vi "loadDataNodeBegin.vi"(8 "error in (no error)":errorcluster, 10 "XML Refnum in":refnum<file>, 11 "FPGADMAChannelData in":refnum<class "FPGADMAChannelData.lvclass">) -> (0 "error out":errorcluster, 2 "XML Refnum out":refnum<file>, 3 "FPGADMAChannelData out":refnum<class "FPGADMAChannelData.lvclass">)   [LabVIEW 2013, in "FPGADMAChannelData.lvclass"]
doc: "Part of the file loading process. Occurs at the beginning of a node being loaded. Loads the common xceDataNode data name and description."
uses:
  FPGADMAChannelData.lvclass
  FPGADMAChannelData.lvclass/FPGADMAChannelData.ctl
  xCE/xceNode/xceNode.lvclass
  XML Parser/XML Parser.lvclass
panel:
  out "text":string[](array[string])
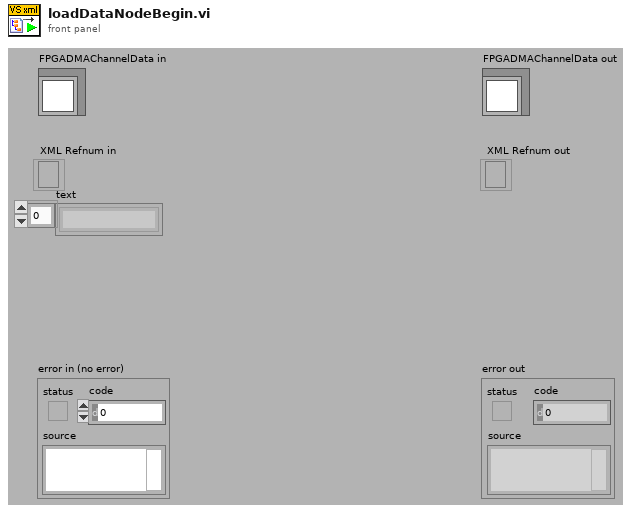
[diagram p1: front panel]
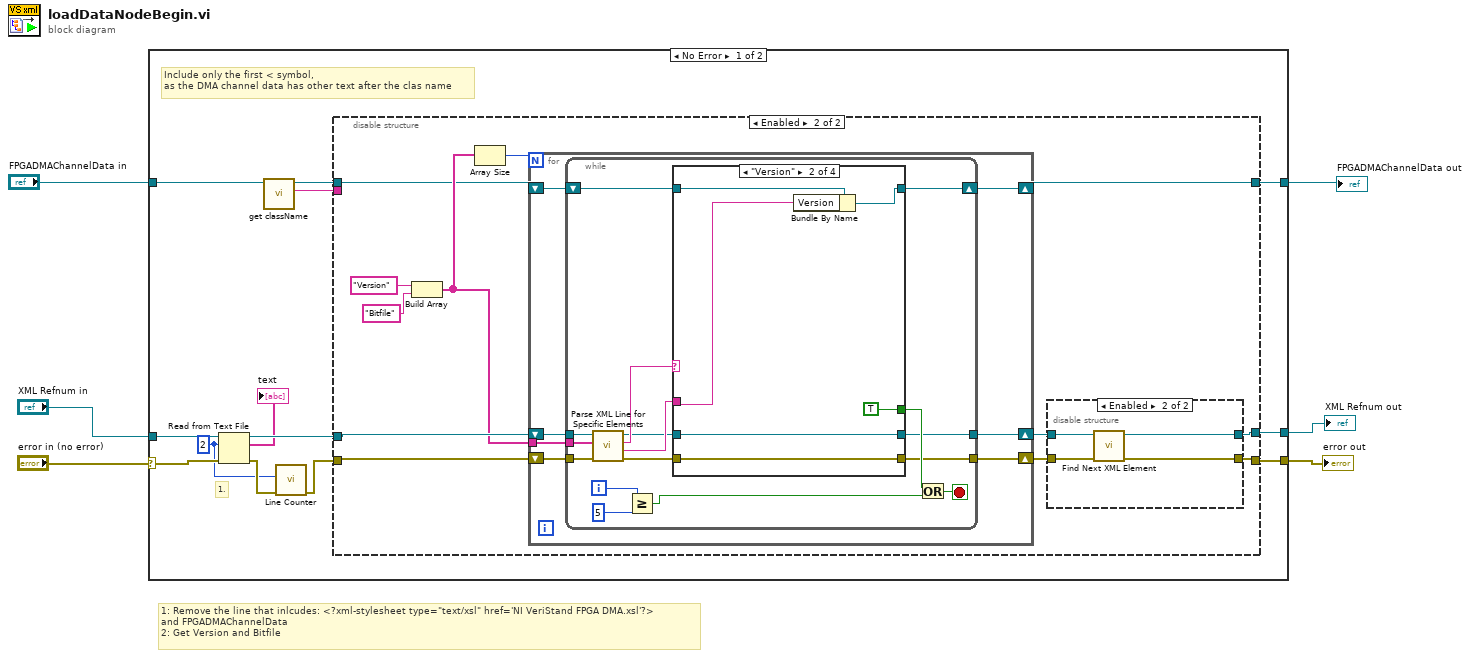
[diagram p0: block diagram]
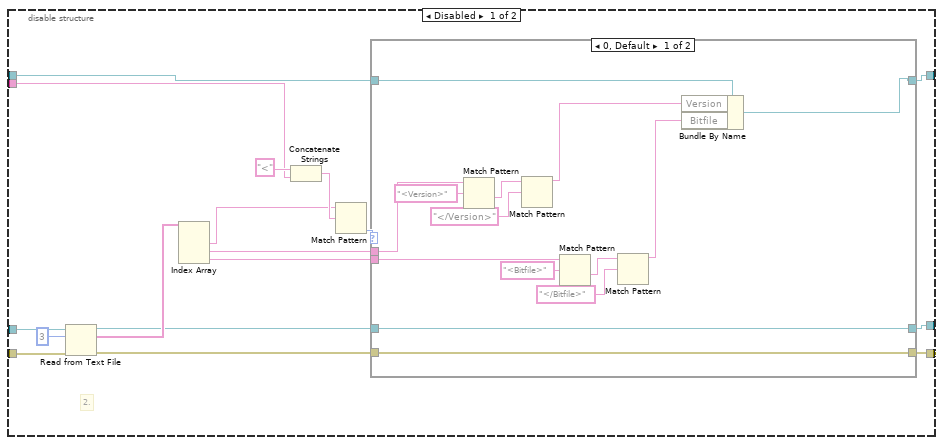
[diagram p2: hidden frame]
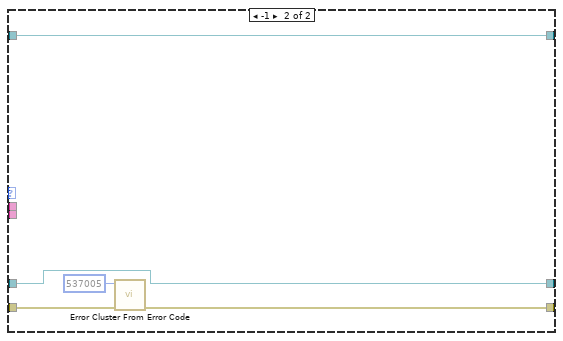
[diagram p3: hidden frame]
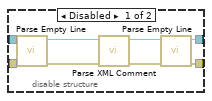
[diagram p4: hidden frame]
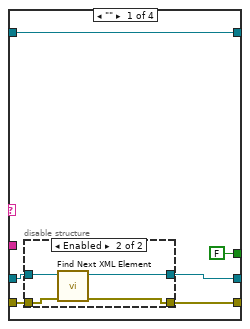
[diagram p5: hidden frame]
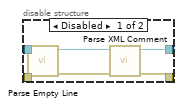
[diagram p6: hidden frame]
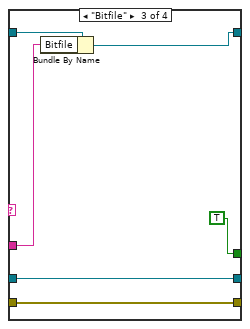
[diagram p7: hidden frame]
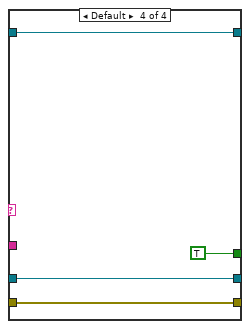
[diagram p8: hidden frame]
diagram:
  # "1: Remove the line that inlcudes: <?xml-stylesheet type=\"text/xsl\" href='NI VeriStand FPGA DMA.xsl'?>\nand FPGADMAChannelData \n2: Get Version and Bitfile"
  n1 = case shown="No Error" "error in (no error)" {
    selector: "error in (no error)" -> [w13 w137]
    tunnel: [w18 w137] -> w3
    tunnel: [w15 w136] -> w2
    tunnel: [w16 w135] -> w1
    tunnel: "FPGADMAChannelData in" -> [w14 w136]
    tunnel: "XML Refnum in" -> [w12 w135]
    frame No Error {
      w7 = 2 ("count")
      # "Include only the first < symbol,\nas the DMA channel data has other text after the clas name"
      # "1."
      n2 = Read from Text File(file (use dialog)=w12, count=w7, error in=w13) -> (refnum out=w11:refnum<file>, text=→"text":string[], error out=w9:errorcluster)  [unwired: 1 in, 1 out]
      n3 = call "get className.vi"("xceNode in"=w14) -> ("Class name"=w19:string, "xceNode out"=w17:refnum<class "FPGADMAChannelData.lvclass">)  [unwired: 8 in, 1 out]
      n4 = call "Line Counter.vi"("error in (no error)"=w9, "# of lines to increment (1)"=w7) -> ("error out"=w8:errorcluster)  [unwired: 8 in, 1 out]
      n5 = disable-structure shown="Enabled" {
        disable-tunnel: w19 -> [w33 _]
        disable-tunnel: [w28 w56] -> w18
        disable-tunnel: w17 -> [w27 w61]
        disable-tunnel: [w23 w57] -> w16
        disable-tunnel: [w22 w60] -> w15
        disable-tunnel: w11 -> [w21 w65]
        disable-tunnel: w8 -> [w20 w64]
        frame Disabled {
          # "2."
          n6 = Read from Text File(file (use dialog)=w21, count=3, error in=w20) -> (refnum out=w24:refnum<file>, text=w35:string[], error out=w30:errorcluster)  [unwired: 1 in, 1 out]
          n7 = Index Array(array=w35) -> (element #1=w31:string, element #2=w26:string, element #3=w25:string)  [unwired: 3 in]
          n8 = Concatenate Strings("<", w33) -> (w32:string)
          n9 = Match Pattern(string=w31, regular expression=w32) -> (offset past match=w29:i32)  [unwired: 1 in, 3 out]
          n10 = case shown="0, Default" w29 {
            tunnel: w30 -> [w50 w55]
            tunnel: [w50 w54] -> w28
            tunnel: w27 -> [w38 w51]
            tunnel: w26 -> [w48 _]
            tunnel: w25 -> [w40 _]
            tunnel: w24 -> [w49 w52]
            tunnel: [w49 w52] -> w23
            tunnel: [w37 w51] -> w22
            frame 0, Default {
              n11 = Match Pattern(string=w48, regular expression="<Version>") -> (after substring=w46:string)  [unwired: 1 in, 3 out]
              n12 = Match Pattern(string=w46, regular expression="</Version>") -> (before substring=w44:string)  [unwired: 1 in, 3 out]
              n13 = Match Pattern(string=w40, regular expression="<Bitfile>") -> (after substring=w42:string)  [unwired: 1 in, 3 out]
              n14 = Match Pattern(string=w42, regular expression="</Bitfile>") -> (before substring=w39:string)  [unwired: 1 in, 3 out]
              n15 = Bundle By Name(cluster=w38, "Version"=w44, "Bitfile"=w39) -> (w37:refnum<class "FPGADMAChannelData.lvclass">)
            }
            frame -1 {
              n16 = call <vilib>:"Error Cluster From Error Code.vi"("error in (no error)"=w55, "error code (0)"=537005) -> ("error out"=w54:errorcluster)  [unwired: 7 in]
            }
          }
        }
        frame Enabled {
          n17 = Build Array("Version" ("regular expression"), "Bitfile" ("regular expression")) -> (w63:string[])
          n18 = Array Size(array=w63) -> (size(s)=w62:i32)
          n19 = for {
            N: w62 -> [_]
            tunnel: w63 -> [w86]
            shift-right: [w81] -> w60
            shift-left: w61 -> [w83]
            shift-right: [w82] -> w59
            shift-left: w65 -> [w85]
            shift-right: [w80] -> w58
            shift-left: w64 -> [w84]
            n20 = while {
              tunnel: w86 -> [w102]
              tunnel: w85 -> [w101]
              tunnel: w84 -> [w100]
              shift-right: [w95] -> w81
              shift-left: w83 -> [w97]
              tunnel: [w87] -> w82
              tunnel: [w88] -> w80
              i -> [w99]
              stop <- w92 stop-if-true
              n21 = call "Parse XML Line for Specific Elements.vi"("error in (no error)"=w100, "Elements"=w102, "XML Refnum in"=w101) -> ("error out"=w89:errorcluster, "Value"=w91:string, "Element Name"=w96:string, "XML Refnum out"=w90:refnum<file>)  [unwired: 4 in, 1 out]
              n22 = Greater Or Equal?(x=w99, y=5) -> (x >= y?=w93:bool)
              n23 = case shown="\"Version\"" w96 {
                tunnel: w97 -> [w108 w124 w130 w134]
                tunnel: [w108 w123 w129 w134] -> w95
                tunnel: [FALSE TRUE TRUE TRUE] -> w94
                tunnel: w91 -> [_ w122 w128 _]
                tunnel: w90 -> [w107 w120 w126 w132]
                tunnel: w89 -> [w106 w119 w125 w131]
                tunnel: [w105 w119 w125 w131] -> w88
                tunnel: [w104 w120 w126 w132] -> w87
                frame "" {
                  n24 = disable-structure shown="Enabled" {
                    disable-tunnel: w107 -> [w114 w118]
                    disable-tunnel: w106 -> [w113 w117]
                    disable-tunnel: [w110 w116] -> w105
                    disable-tunnel: [w109 w115] -> w104
                    frame Disabled {
                      n25 = call "Parse Empty Line.vi"("error in (no error)"=w113, "XML Refnum in"=w114) -> ("error out"=w111:errorcluster, "XML Refnum out"=w112:refnum<file>)  [unwired: 7 in, 1 out]
                      n26 = call "Parse XML Comment.vi"("error in (no error)"=w111, "XML Refnum in"=w112) -> ("error out"=w110:errorcluster, "XML Refnum out"=w109:refnum<file>)  [unwired: 6 in, 2 out]
                    }
                    frame Enabled {
                      n27 = call "Find Next XML Element.vi"("error in (no error)"=w117, "XML Fine In"=w118) -> ("error out"=w116:errorcluster, "XML Fine Out"=w115:refnum<file>)  [unwired: 7 in, 1 out]
                    }
                  }
                }
                frame "Version" {
                  n28 = Bundle By Name(cluster=w124, "Version"=w122) -> (w123:refnum<class "FPGADMAChannelData.lvclass">)
                }
                frame "Bitfile" {
                  n29 = Bundle By Name(cluster=w130, "Bitfile"=w128) -> (w129:refnum<class "FPGADMAChannelData.lvclass">)
                }
                frame Default {
                }
              }
              n30 = Or(x=w94, y=w93) -> (x .or. y?=w92:bool)
            }
          }
          n31 = disable-structure shown="Enabled" {
            disable-tunnel: w59 -> [w71 w79]
            disable-tunnel: w58 -> [w70 w77]
            disable-tunnel: [w69 w78] -> w57
            disable-tunnel: [w68 w76] -> w56
            frame Disabled {
              n32 = call "Parse Empty Line.vi"("error in (no error)"=w70, "XML Refnum in"=w71) -> ("error out"=w74:errorcluster, "XML Refnum out"=w75:refnum<file>)  [unwired: 7 in, 1 out]
              n33 = call "Parse XML Comment.vi"("error in (no error)"=w74, "XML Refnum in"=w75) -> ("error out"=w72:errorcluster, "XML Refnum out"=w73:refnum<file>)  [unwired: 6 in, 2 out]
              n34 = call "Parse Empty Line.vi"("error in (no error)"=w72, "XML Refnum in"=w73) -> ("error out"=w68:errorcluster, "XML Refnum out"=w69:refnum<file>)  [unwired: 7 in, 1 out]
            }
            frame Enabled {
              n35 = call "Find Next XML Element.vi"("error in (no error)"=w77, "XML Fine In"=w79) -> ("error out"=w76:errorcluster, "XML Fine Out"=w78:refnum<file>)  [unwired: 7 in, 1 out]
            }
          }
        }
      }
    }
    frame Error {
    }
  }
  "error out" <- w3
  "FPGADMAChannelData out" <- w2
  "XML Refnum out" <- w1
